vi "Параллельный регистр(4-разрядный).vi"(1 "C":bool, 2 "Reset":bool, 3 "Cluster":T2) -> (0 "output cluster":T1)   [LabVIEW 2013]
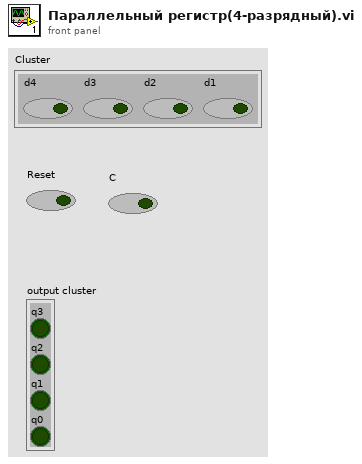
[diagram p1: front panel]
types:
  T1 = cluster{"q3":bool, "q2":bool, "q1":bool, "q0":bool}
  T2 = cluster{"d4":bool, "d3":bool, "d2":bool, "d1":bool}
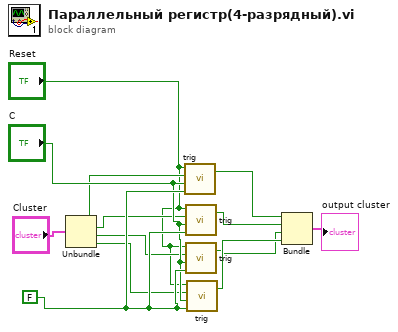
[diagram p0: block diagram]
diagram:
  w12 = FALSE
  n1 = Unbundle("Cluster") -> ("d4"=w7:bool, "d3"=w8:bool, "d2"=w9:bool, "d1"=w10:bool)
  n2 = call "trig.vi"("s"=w12, "c"="C", "d"=w7, "r"="Reset") -> ("q"=w2:bool)  [unwired: 1 out]
  n3 = call "trig.vi"("s"=w12, "c"="C", "d"=w8, "r"="Reset") -> ("q"=w3:bool)  [unwired: 1 out]
  n4 = call "trig.vi"("s"=w12, "c"="C", "d"=w9, "r"="Reset") -> ("q"=w4:bool)  [unwired: 1 out]
  n5 = call "trig.vi"("s"=w12, "c"="C", "d"=w10, "r"="Reset") -> ("q"=w5:bool)  [unwired: 1 out]
  n6 = Bundle("q"=w2, "q"=w3, "q"=w4, "q"=w5) -> (→"output cluster":cluster{"q":bool, "q":bool, "q":bool, "q":bool})  [unwired: 1 in]
